vi "Convert Farrads to Num.vi"(1 "Numeric":dbl) -> (0 "String":string)   [LabVIEW 2013]
panel:
  out "number":u32
  out "Numeric (SI Notation)":dbl format="%#_6p"
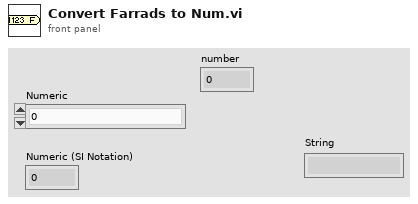
[diagram p1: front panel]
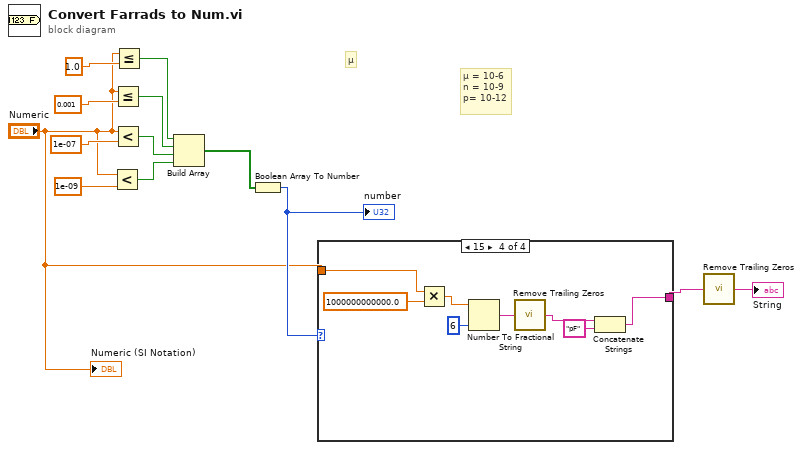
[diagram p0: block diagram]
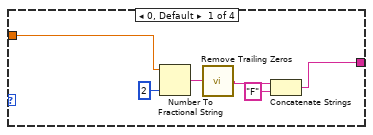
[diagram p2: hidden frame]
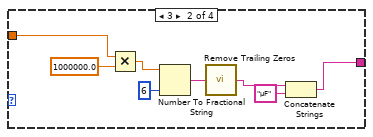
[diagram p3: hidden frame]
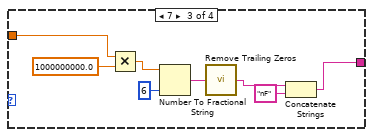
[diagram p4: hidden frame]
diagram:
  # "µ = 10-6\nn = 10-9\np= 10-12"
  # "µ"
  n1 = Less?(x="Numeric", y=1e-09) -> (x < y?=w7:bool)
  n2 = Less Or Equal?(x="Numeric", y=0.001) -> (x <= y?=w4:bool)
  n3 = Less?(x="Numeric", y=1e-07) -> (x < y?=w8:bool)
  n4 = Less Or Equal?(x="Numeric", y=1.0) -> (x <= y?=w1:bool)
  n5 = Build Array(w1, w4, w8, w7) -> (w6:bool[])
  n6 = Boolean Array To Number(Boolean array=w6) -> (number=w13:u32)
  "number" <- w13
  n7 = case shown="15" w13 {
    tunnel: [w18 w26 w34 w42] -> w12
    tunnel: "Numeric" -> [w17 w22 w30 w38]
    frame 0, Default {
      n8 = Number To Fractional String(number=w17, precision (6)=i16 2) -> (F-format string=w15:string)  [unwired: 2 in]
      n9 = call "Remove Trailing Zeros.vi"("String In"=w15) -> ("String Out"=w14:string)
      n10 = Concatenate Strings(w14, "F" ("string")) -> (w18:string)
    }
    frame 3 {
      n11 = Multiply(x=w22, y=1000000.0) -> (x*y=w21:dbl)
      n12 = Number To Fractional String(number=w21, precision (6)=i16 6) -> (F-format string=w24:string)  [unwired: 2 in]
      n13 = call "Remove Trailing Zeros.vi"("String In"=w24) -> ("String Out"=w23:string)
      n14 = Concatenate Strings(w23, "µF" ("string")) -> (w26:string)
    }
    frame 7 {
      n15 = Multiply(x=w30, y=1000000000.0) -> (x*y=w29:dbl)
      n16 = Number To Fractional String(number=w29, precision (6)=i16 6) -> (F-format string=w32:string)  [unwired: 2 in]
      n17 = call "Remove Trailing Zeros.vi"("String In"=w32) -> ("String Out"=w31:string)
      n18 = Concatenate Strings(w31, "nF" ("string")) -> (w34:string)
    }
    frame 15 {
      n19 = Multiply(x=w38, y=1000000000000.0) -> (x*y=w37:dbl)
      n20 = Number To Fractional String(number=w37, precision (6)=i16 6) -> (F-format string=w40:string)  [unwired: 2 in]
      n21 = call "Remove Trailing Zeros.vi"("String In"=w40) -> ("String Out"=w39:string)
      n22 = Concatenate Strings(w39, "pF" ("string")) -> (w42:string)
    }
  }
  n23 = call "Remove Trailing Zeros.vi"("String In"=w12) -> ("String Out"=→"String":string)
  "Numeric (SI Notation)" <- "Numeric"
